vi "Double FFT Mesurament (Max Bin detection - Control) test.vi"() -> ()   [LabVIEW 2014]
uses:
  <vilib>/Platform/TimedLoop/XDataNode/timing_clust.ctl
  <vilib>/Platform/TimedLoop/XDataNode/nitl_modes.ctl
  <vilib>/Platform/TimedLoop/XDataNode/wakeup.ctl
  <vilib>/rvi/Analysis/measure/FFT/simModelSupport/niFPGA FFT Streaming Sim Properties.ctl
  <vilib>/rvi/Analysis/measure/FFT/simModelSupport/niFPGA FFT Sim Stream Group Properties.ctl
  <vilib>/rvi/Analysis/measure/FFT/simModelSupport/niFPGA FFT Sim Types.ctl
  <vilib>/rvi/Analysis/measure/FFT/simModelSupport/niFpgaFFTSimArithmeticProperties.ctl
  <vilib>/rvi/Analysis/measure/FFT/simModelSupport/niFpgaFFTSimDfxp.ctl
  <vilib>/fxp/LVFixedPointQuantizationPolicyTypeDef.ctl
  <vilib>/rvi/Analysis/measure/FFT/XNode/niFpgaFFTButterflyDelays.ctl
  <vilib>/rvi/Emulation/niFpgaSctlEmulationGetInTimedLoop.vi
  <vilib>/rvi/Emulation/niFpgaEmulationReportErrorSimple.vi
  <vilib>/rvi/Emulation/niFpgaGetClockAttributes.vi
  <vilib>/rvi/Emulation/niFpgaCriticalErrorInLSC.vi
  <vilib>/rvi/Emulation/niFpgaEmulationIsFPGAContextNoSignature.vi
  <vilib>/rvi/errors/niFpgaSetErrorForExecOnDevCompSimple.vi
  <vilib>/rvi/eio/common/nirviEmuReportErrorAndStop.vi
  <vilib>/rvi/DataTransferAndStorage/Container/Common/niFpgaContainerGetUniqueNameForEmu.vi
  <vilib>/rvi/FIFO/Fifo_Resource/nirvififoEmulationSetSize.vi
  <vilib>/rvi/FIFO/Fifo_Resource/nirviFifoEmulationQueueMgr.vi
  <instcachedir>/0/nirviFifoEmulationQueueMgr_E5CAEC123FF24DC58D834DCA3CDAA9B5.lvgen/nirviFifoEmulationQueueMgr_E5CAEC123FF24DC58D834DCA3CDAA9B5_012.vi
  <vilib>/rvi/FIFO/Fifo_Resource/nirvififoEmulationCreateLock.vi
  <vilib>/rvi/Emulation/niFpgaProcessEmulError.vi
  <vilib>/rvi/FIFO/Fifo_Resource/nirvififoEmulationObtainLock.vi
  <vilib>/rvi/FIFO/Fifo_Resource/nirvififoEmulationReleaseLock.vi
  <vilib>/rvi/occurrence/nirviWaitOnOccurrenceBase.vi
  <vilib>/rvi/errors/nirviReportUnexpectedCaseInternalError.vi
  <vilib>/rvi/errors/nirviReportUnexpectedCaseInternalError (U32).vi
  <vilib>/rvi/Memory/Memory_Emulation/niFpgaMemoryEmulationCacheClearOnFirstRun.vi
  <vilib>/rvi/Memory/Memory_Emulation/nirvimemoryEmulationManagerCache_MakeExclusive.vi
  <vilib>/rvi/Memory/Memory_Emulation/niFpgaMemoryEmulationValidateCache.vi
  <vilib>/rvi/Memory/Memory_Emulation/nirvimemoryEmulationManagerCache_InsertValue.vi
  <vilib>/Utility/error.llb/Clear Errors.vi
  <vilib>/rvi/Memory/Memory_Emulation/nirvimemoryEmulationManagerCache_ReleaseExclusive.vi
  <vilib>/rvi/Memory/Memory_Emulation/nirvimemoryEmulationManagerCache_GetValue.vi
  <vilib>/rvi/Memory/Memory_Emulation/nirvimemoryEmulationManagerCache_SetValue.vi
  <instcachedir>/0/nirviFifoEmulationQueueMgr_E5CAEC123FF24DC58D834DCA3CDAA9B5.lvgen/nirviFifoEmulationQueueMgr_E5CAEC123FF24DC58D834DCA3CDAA9B5_010.vi
  <vilib>/rvi/FIFO/Fifo_Resource/nirvififoEmulationDetermineInputValidOut.vi
  <vilib>/rvi/Memory/Memory_Emulation/nirvimemoryFastEmulation.vi
  <vilib>/rvi/Memory/Memory_Emulation/nirvimemoryEmulation.vi
  <vilib>/rvi/Analysis/measure/FFT/simModelSupport/niFpgaFFTSimModelStreamingCore.vi
  <vilib>/rvi/eio/common/nirviEmuTemplateMethod_errors.vi
  <vilib>/Platform/TimedLoop/XDataNode/XDataNode.xnode
  <vilib>/rvi/DataTransferAndStorage/Container/XNode/niFpgaContainer.xnode
  <vilib>/rvi/FIFO/Fifo_Resource/nirvififoEmulationRead.vi
  <vilib>/rvi/DataTransferAndStorage/Register/Emulation/niFpgaRegisterEmulation.vi
  <vilib>/rvi/FIFO/Fifo_Resource/nirvififoEmulationWrite.vi
  <vilib>/rvi/FIFO/Fifo_Resource/nirvififoEmulationGetNumberOfElementsToWrite.vi
  <vilib>/rvi/Analysis/measure/FFT/XNode/niFpgaFFT.xnode
  <vilib>/eio/EIOMethodNode/EIOMethodNode.xnode
  <vilib>/Platform/TimedLoop/XDataNode/XDNodeRunTimeDep.lvlib
panel:
  in  "first bin":i32=4
  in  "last bin":i32=251
  in  "lower limit 2":u32=682
  in  "lower limit 1":u32=57
  in  "upper limit 2":u32=1194
  in  "upper limit 1":u32=569
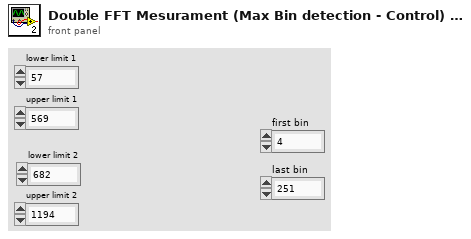
[diagram p1: front panel]
types:
  T1 = typedef "XDNodeRunTimeDep.lvlib/timing_clust.ctl" = cluster{"Expected End [f-1]":u64, "Actual End [f-1]":u64, "Finished Late? [f-1]":bool, "Expected End [i-1]":u64, "Actual End [i-1]":u64, "Finished Late? [i-1]":bool, "Expected Start [i]":u64, "Actual Start [i]":u64, "Expected Start [f]":u64, "Actual Start [f]":u64, "Source Name":string, "Structure Name":string, "Period":i64, "Deadline":i64, "Offset":i64, "Start":i64, "Priority":i32, "Timeout":i32, "Mode":T2, "Wakeup Reason":T3, "Error":errorcluster, "Source Type":string, "Secondary Source Type":string, "Global End Time":u64, "Global Start Time":u64, "Frame Duration":u64, "Iteration Duration":u64, "Assigned CPU":i32, "I/O Scan Engine Mode":u32}
  T2 = typedef "XDNodeRunTimeDep.lvlib/nitl_modes.ctl" = enum32{"No Change", "Process missed periods, maintain original phase", "Discard missed periods, maintain original phase", "Process missed periods, ignore original phase", "Discard missed periods, ignore original phase"}
  T3 = typedef "XDNodeRunTimeDep.lvlib/wakeup.ctl" = enum32{"Normal", "Aborted", "Asynchronous wakeup", "Timing source error", "Timed loop error", "Timeout"}
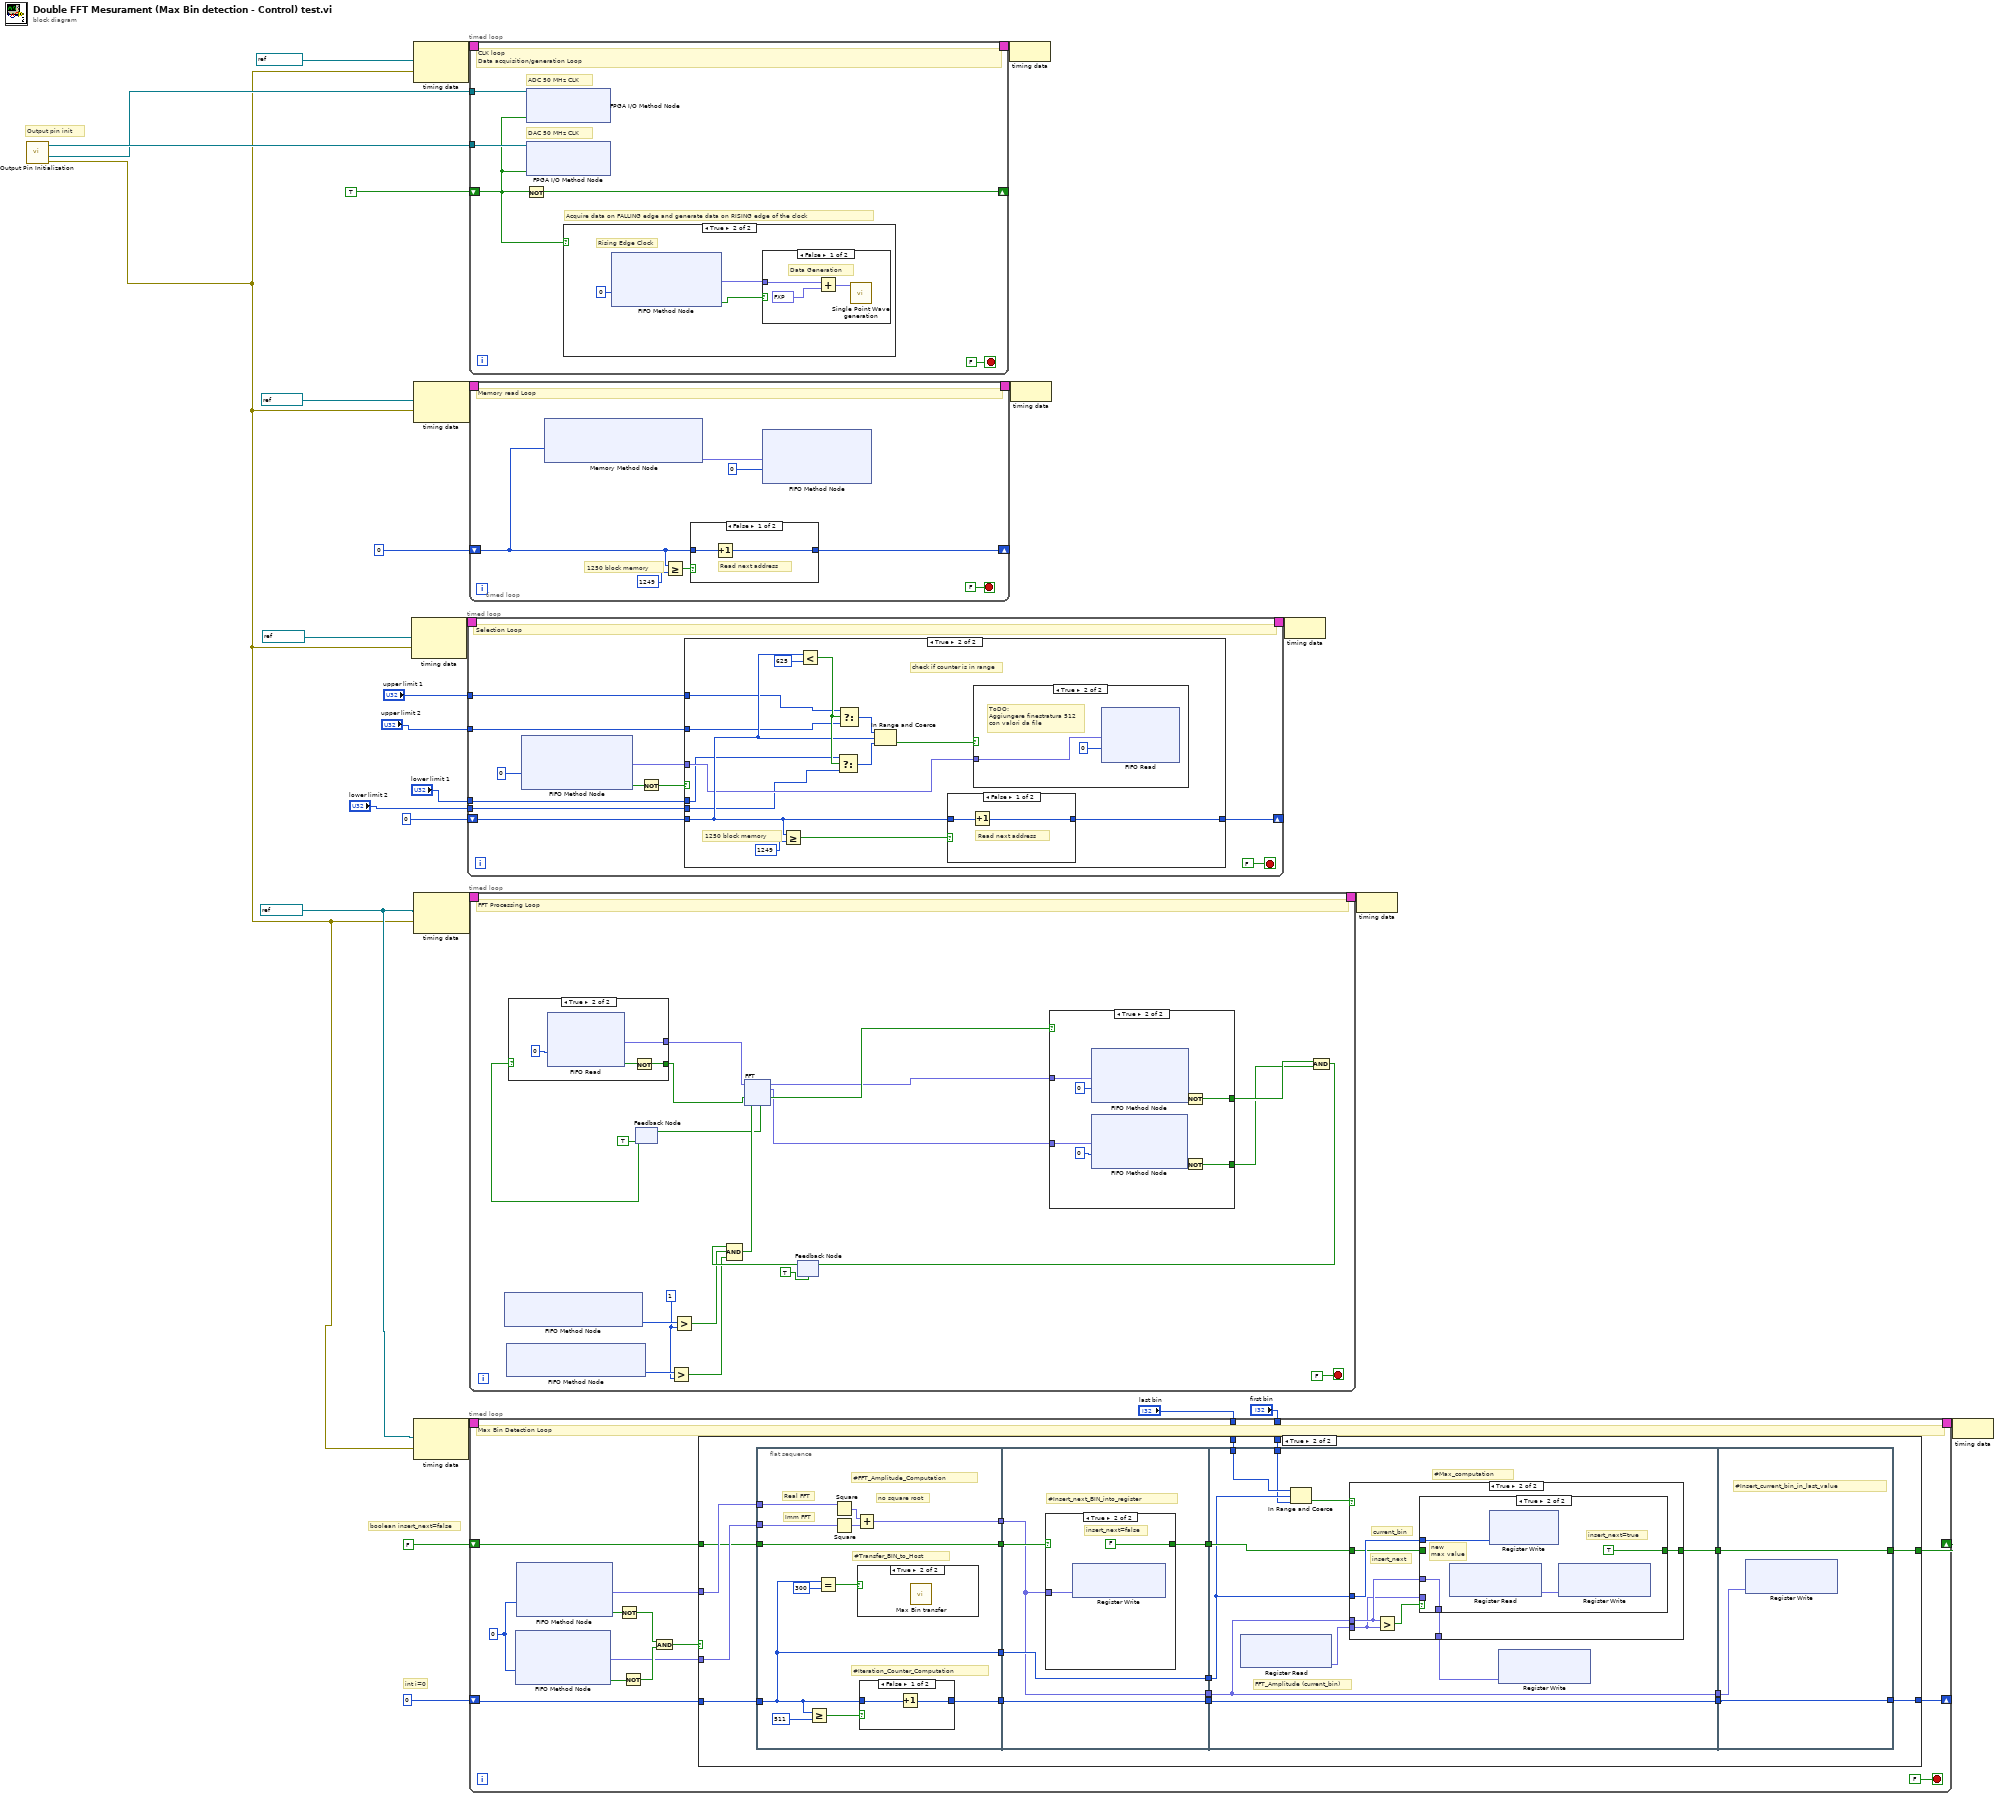
[diagram p0: block diagram]
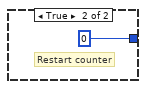
[diagram p4: hidden frame]
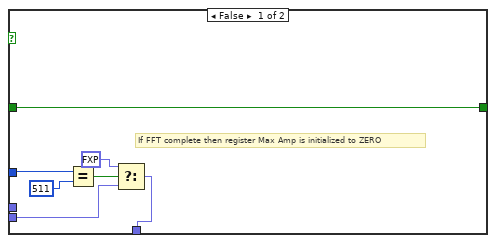
[diagram p6: hidden frame]
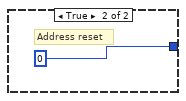
[diagram p10: hidden frame]
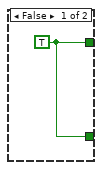
[diagram p11: hidden frame]
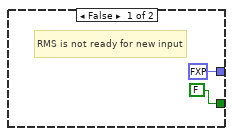
[diagram p12: hidden frame]
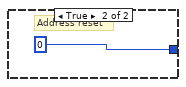
[diagram p13: hidden frame]
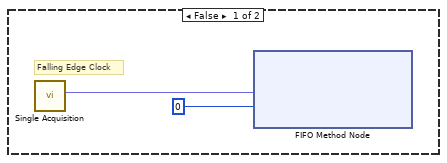
[diagram p14: hidden frame]
diagram:
  w8 = refnum<k21> "50MHz" ("Source Name")
  # "int i=0"
  # "boolean insert_next=false"
  # "Output pin init"
  n1 = call "Output Pin Initialization.vi"() -> ("error out"=w7:errorcluster, "I/O Out Clock DAC (pin16)"=w15:refnum<k21>, "I/O Out Clock ADC (pin17)"=w16:refnum<k21>)  [unwired: 8 in]
  n2 = node-c288(refnum<k21> "50MHz" ("Source Name"), w7) -> (w22:T1)
  n3 = node-c288(refnum<k21> "100MHz" ("Source Name"), w7) -> (w28:T1)
  n4 = node-c288(w8, w7) -> (w10:T1)
  n5 = node-c288(refnum<k21> "50MHz" ("Source Name"), w7) -> (w26:T1)
  n6 = node-c288(w8, w7) -> (w24:T1)
  n7 = timed-loop {
    timing: w22 -> [_]
    timing-out: [_] -> w21
    shift-right: [w38] -> _
    shift-left: u32 0 -> [w37]
    tunnel: "upper limit 1" -> [w32]
    tunnel: "upper limit 2" -> [w31]
    tunnel: "lower limit 1" -> [w30]
    tunnel: "lower limit 2" -> [w29]
    stop <- FALSE stop-if-true
    # "Selection Loop"
    n8 = xnode ("FIFO Method Node")("Timeout"=0) -> ("Element"=w34:fxp<+/-,12,12>, "Timed Out?"=w35:bool)  [unwired: 1 in, 1 out]
    n9 = Not(x=w35) -> (.not. x?=w36:bool)
    n10 = case shown="True" w36 {
      tunnel: [w40 w52] -> w38
      tunnel: w37 -> [w40 w47]
      tunnel: w34 -> [_ w45]
      tunnel: w32 -> [_ w44]
      tunnel: w31 -> [_ w43]
      tunnel: w30 -> [_ w42]
      tunnel: w29 -> [_ w41]
      frame False {
      }
      frame True {
        # "check if counter is in range"
        # "1250 block memory"
        n11 = Greater Or Equal?(x=w47, y=u32 1249) -> (x >= y?=w53:bool)
        n12 = Less?(x=w47, y=u32 625) -> (x < y?=w48:bool)
        n13 = Select(t=w42, s=w48, f=w41) -> (s? t:f=w50:u32)
        n14 = Select(t=w44, s=w48, f=w43) -> (s? t:f=w51:u32)
        n15 = In Range and Coerce(upper limit=w51, x=w47, lower limit=w50) -> (In Range?=w46:bool)  [unwired: 1 out]
        n16 = case shown="False" w53 {
          tunnel: w47 -> [w58 _]
          tunnel: [w57 u32 0] -> w52
          frame False {
            # "Read next address"
            n17 = Increment(x=w58) -> (x+1=w57:u32)
          }
          frame True {
            # "Address reset"
          }
        }
        n18 = case shown="True" w46 {
          tunnel: w45 -> [_ w56]
          frame False {
          }
          frame True {
            # "ToDO:\nAggiungere finestratura 512\ncon valori da file"
            n19 = xnode ("FIFO Read")("Element"=w56, "Timeout"=0) -> ()  [unwired: 1 in, 2 out]
          }
        }
      }
    }
  }
  n20 = timed-loop {
    timing: w28 -> [_]
    timing-out: [_] -> w27
    shift-right: [w64] -> _
    shift-left: TRUE -> [w62]
    tunnel: w15 -> [w66]
    tunnel: w16 -> [w63]
    stop <- FALSE stop-if-true
    # "DAC 50 MHz CLK"
    # "Acquire data on FALLING edge and generate data on RISING edge of the clock"
    # "ADC 50 MHz CLK"
    # "CLK loop\nData acquisition/generation Loop"
    n21 = Not(x=w62) -> (.not. x?=w64:bool)
    n22 = xnode "FPGA I/O Method Node"("FPGA I/O In"=w66, "Data"=w62) -> ()  [unwired: 1 out]
    n23 = xnode "FPGA I/O Method Node"("FPGA I/O In"=w63, "Data"=w62) -> ()  [unwired: 1 out]
    n24 = case shown="True" w62 {
      frame False {
        # "Falling Edge Clock"
        n25 = call "Single Acquisition.vi"() -> ("Out"=w68:fxp<+/-,12,12>)  [unwired: 10 in, 1 out]
        n26 = xnode ("FIFO Method Node")("Element"=w68, "Timeout"=0) -> ()  [unwired: 1 in, 2 out]
      }
      frame True {
        # "Rising Edge Clock"
        n27 = xnode ("FIFO Method Node")("Timeout"=0) -> ("Element"=w69:fxp<+/-,12,12>, "Timed Out?"=w70:bool)  [unwired: 1 in, 1 out]
        n28 = case shown="False" w70 {
          tunnel: w69 -> [w74 _]
          frame False {
            # "Data Generation"
            n29 = Add(x=w74, y=fxp<+,12,12> 2048.0) -> (x+y=w72:fxp<+/-,14,14>)
            n30 = call "Single Point Wave generation.vi"("Data To Write"=w72) -> ()  [unwired: 10 in, 1 out]
          }
          frame True {
            # "FPGA memory slow"
          }
        }
      }
    }
  }
  n31 = timed-loop {
    shift-right: [w82] -> _
    shift-left: 0 ("Timeout") -> [w83]
    shift-right: [w80] -> _
    shift-left: FALSE -> [w81]
    timing: w10 -> [_]
    timing-out: [_] -> w9
    tunnel: "last bin" -> [w78]
    tunnel: "first bin" -> [w77]
    stop <- FALSE stop-if-true
    w91 = 0 ("Timeout")
    # "Max Bin Detection Loop"
    n32 = xnode ("FIFO Method Node")("Timeout"=w91) -> ("Element"=w84:fxp<+/-,22,22>, "Timed Out?"=w89:bool)  [unwired: 1 in, 1 out]
    n33 = xnode ("FIFO Method Node")("Timeout"=w91) -> ("Element"=w85:fxp<+/-,22,22>, "Timed Out?"=w90:bool)  [unwired: 1 in, 1 out]
    n34 = Not(x=w90) -> (.not. x?=w88:bool)
    n35 = Not(x=w89) -> (.not. x?=w87:bool)
    n36 = And(x=w88, y=w87) -> (x .and. y?=w86:bool)
    n37 = case shown="True" w86 {
      tunnel: w85 -> [_ w112]
      tunnel: w84 -> [_ w111]
      tunnel: w83 -> [w93 w109]
      tunnel: [w93 w96] -> w82
      tunnel: w81 -> [w92 w103]
      tunnel: [w92 w98] -> w80
      tunnel: w78 -> [_ w95]
      tunnel: w77 -> [_ w94]
      frame False {
        # "Data are NOT ready in Target Real FFT and Target Imm FFT FIFOs"
      }
      frame True {
        n38 = flat-sequence {
          tunnel: w112 -> [w121]
          tunnel: w111 -> [w122]
          tunnel: [w120] -> w110
          tunnel: w109 -> [w113]
          tunnel: [w119] -> w108
          tunnel: [w113] -> w105
          tunnel: [w116] -> w104
          tunnel: w103 -> [w116]
          tunnel: w110 -> [w129]
          tunnel: w108 -> [w132]
          tunnel: [w132] -> w107
          tunnel: w105 -> [w130]
          tunnel: w104 -> [w131]
          tunnel: [w130] -> w102
          tunnel: [w129] -> w101
          tunnel: [w128] -> w100
          tunnel: w107 -> [w145]
          tunnel: [w145] -> w106
          tunnel: w102 -> [w140]
          tunnel: w101 -> [w142]
          tunnel: w100 -> [w143]
          tunnel: [w142] -> w99
          tunnel: [w141] -> w97
          tunnel: w95 -> [w137]
          tunnel: w94 -> [w136]
          tunnel: w106 -> [w166]
          tunnel: w99 -> [w168]
          tunnel: w97 -> [w167]
          tunnel: [w167] -> w98
          tunnel: [w166] -> w96
          frame #0 {
            # "no square root"
            # "#Transfer_BIN_to_Host"
            # "#Iteration_Counter_Computation"
            # "#FFT_Amplitude_Computation"
            # "Imm FFT"
            # "Real FFT"
            n39 = Greater Or Equal?(x=w113, y=511) -> (x >= y?=w117:bool)
            n40 = Equal?(x=w113, y=300) -> (x = y?=w115:bool)
            n41 = Square(x=w121) -> (x^2=w124:fxp<+,43,43>)
            n42 = Square(x=w122) -> (x^2=w123:fxp<+,43,43>)
            n43 = Add(x=w124, y=w123) -> (x+y=w120:fxp<+,44,44>)
            n44 = case shown="True" w115 {
              frame False {
                # "FFT Comp is NOT finished"
              }
              frame True {
                n45 = call "Max Bin transfer.vi"() -> ()  [unwired: 11 in, 1 out]
              }
            }
            n46 = case shown="False" w117 {
              tunnel: w113 -> [w125 _]
              tunnel: [w126 0 ("Timeout")] -> w119
              frame False {
                n47 = Increment(x=w125) -> (x+1=w126:i32)
              }
              frame True {
                # "Restart counter"
              }
            }
          }
          frame #1 {
            # "#Insert_next_BIN_into_register"
            n48 = case shown="True" w131 {
              selector: w131 -> [w133 _]
              tunnel: [w133 FALSE] -> w128
              tunnel: w129 -> [_ w134]
              frame False {
              }
              frame True {
                # "insert_next=false"
                n49 = xnode ("Register Write")("Data"=w134) -> ()  [unwired: 1 in, 1 out]
              }
            }
          }
          frame #2 {
            # "FFT_Amplitude (current_bin)"
            # "#Max_computation"
            n50 = xnode ("Register Read")() -> ("Data"=w139:fxp<+,44,44>)  [unwired: 1 in, 1 out]
            n51 = In Range and Coerce(upper limit=w137, x=w140, lower limit=w136) -> (In Range?=w144:bool)  [unwired: 1 out]
            n52 = case shown="True" w144 {
              tunnel: w142 -> [_ w158]
              tunnel: w140 -> [w150 w157]
              tunnel: w143 -> [w152 w156]
              tunnel: [w152 w155] -> w141
              tunnel: w139 -> [w148 w153]
              tunnel: [w146 w154] -> w138
              frame False {
                # "If FFT complete then register Max Amp is initialized to ZERO"
                n53 = Equal?(x=w150, y=511) -> (x = y?=w151:bool)
                n54 = Select(t=fxp<+,44,44> 0.0, s=w151, f=w148) -> (s? t:f=w146:fxp<+,44,44>)
              }
              frame True {
                # "insert_next"
                # "current_bin"
                n55 = Greater?(x=w158, y=w153) -> (0:w159:bool)
                n56 = case shown="True" w159 {
                  tunnel: w158 -> [_ w162]
                  tunnel: w157 -> [_ w165]
                  tunnel: w156 -> [w161 _]
                  tunnel: [w161 TRUE] -> w155
                  tunnel: [w160 w162] -> w154
                  tunnel: w153 -> [w160 _]
                  frame False {
                    # "Old value is re-written"
                  }
                  frame True {
                    # "new\nmax value"
                    # "insert_next=true"
                    n57 = xnode ("Register Read")() -> ("Data"=w163:fxp<+,44,44>)  [unwired: 1 in, 1 out]
                    n58 = xnode ("Register Write")("Data"=w165) -> ()  [unwired: 1 in, 1 out]
                    n59 = xnode ("Register Write")("Data"=w163) -> ()  [unwired: 1 in, 1 out]
                  }
                }
              }
            }
            n60 = xnode ("Register Write")("Data"=w138) -> ()  [unwired: 1 in, 1 out]
          }
          frame #3 {
            # "#Insert_current_bin_in_last_value"
            n61 = xnode ("Register Write")("Data"=w168) -> ()  [unwired: 1 in, 1 out]
          }
        }
      }
    }
  }
  n62 = timed-loop {
    timing: w26 -> [_]
    timing-out: [_] -> w25
    shift-right: [w175] -> _
    shift-left: u32 0 -> [w173]
    stop <- FALSE stop-if-true
    # "1250 block memory"
    # "Memory read Loop"
    n63 = xnode ("Memory Method Node")("Address"=w173) -> ("Data"=w172:fxp<+/-,12,12>)  [unwired: 1 in, 1 out]
    n64 = Greater Or Equal?(x=w173, y=u32 1249) -> (x >= y?=w176:bool)
    n65 = case shown="False" w176 {
      tunnel: w173 -> [w179 _]
      tunnel: [w178 u32 0] -> w175
      frame False {
        # "Read next address"
        n66 = Increment(x=w179) -> (x+1=w178:u32)
      }
      frame True {
        # "Address reset"
      }
    }
    n67 = xnode ("FIFO Method Node")("Element"=w172, "Timeout"=0) -> ()  [unwired: 1 in, 2 out]
  }
  n68 = timed-loop {
    timing: w24 -> [_]
    timing-out: [_] -> w23
    stop <- FALSE stop-if-true
    w185 = u32 1 ("y")
    # "FFT Processing Loop"
    n69 = xnode ("FIFO Method Node")() -> ("Number of Elements to Write"=w187:u32)  [unwired: 1 in, 1 out]
    n70 = xnode ("FIFO Method Node")() -> ("Number of Elements to Write"=w186:u32)  [unwired: 1 in, 1 out]
    n71 = feedback #1(TRUE ("ready for input")) -> (w202:bool)
    n72 = case shown="True" w202 {
      tunnel: [FALSE w243] -> w196
      tunnel: [fxp<+/-,12,12> 0.0 ("Element") w240] -> w197
      frame False {
        # "RMS is not ready for new input"
      }
      frame True {
        n73 = xnode ("FIFO Read")("Timeout"=0) -> ("Element"=w240:fxp<+/-,12,12>, "Timed Out?"=w242:bool)  [unwired: 1 in, 1 out]
        n74 = Not(x=w242) -> (.not. x?=w243:bool)
      }
    }
    n75 = Greater?(x=w186, y=w185) -> (0:w183:bool)
    n76 = Greater?(x=w187, y=w185) -> (0:w184:bool)
    n77 = feedback #2(TRUE) -> (w198:bool)
    n78 = Compound Arithmetic op=AND(w198, w184, w183) -> (w195:bool)
    n79 = xnode "FFT"("real data in"=w197, "input valid"=w196, "ready for output"=w195) -> ("ready for input"=w194:bool, "real data out"=w192:fxp<+/-,22,22>, "imaginary data out"=w191:fxp<+/-,22,22>, "output valid"=w193:bool)  [unwired: 2 in, 1 out]
    n80 = feedback-in #1(w194) -> ()
    n81 = case shown="True" w193 {
      tunnel: w192 -> [_ w237]
      tunnel: w191 -> [_ w236]
      tunnel: [w229 w235] -> w190
      tunnel: [w229 w234] -> w189
      frame False {
        w229 = TRUE
      }
      frame True {
        n82 = xnode ("FIFO Method Node")("Element"=w237, "Timeout"=0) -> ("Timed Out?"=w230:bool)  [unwired: 1 in, 1 out]
        n83 = xnode ("FIFO Method Node")("Element"=w236, "Timeout"=0) -> ("Timed Out?"=w231:bool)  [unwired: 1 in, 1 out]
        n84 = Not(x=w230) -> (.not. x?=w235:bool)
        n85 = Not(x=w231) -> (.not. x?=w234:bool)
      }
    }
    n86 = Compound Arithmetic op=AND(w190, w189) -> (w188:bool)
    n87 = feedback-in #2(w188) -> ()
  }
  n88 = node-c288(w27) -> ()
  n89 = node-c288(w25) -> ()
  n90 = node-c288(w21) -> ()
  n91 = node-c288(w23) -> ()
  n92 = node-c288(w9) -> ()
